vi "Tetra_PROD_Instruments.vi"(8 "error in":errorcluster) -> (1 "error out":errorcluster, 3 "This VI":refnum<vi>)   [LabVIEW 2018]
uses:
  <vilib>/Utility/error.llb/DialogType.ctl
  Initialize References/Sequence Globals.vi
  <vilib>/Utility/file.llb/Read Delimited Spreadsheet (string).vi
  Initialize References/Station References Global.vi
  Tetra_Globals.vi
  Instruments/Keysight N9010A/Agilent MXA Series/Agilent MXA Series.lvlib
  Instruments/Agilent N5232A PNA-L/Labview Driver/Keysight PNA Series/Keysight PNA Series.lvlib
panel:
  out "SN_LIST":string[][](array[string])
  out "selected comport":string
  out "USB toSER Present?":bool=TRUE
  out "find list":string[](array[string])
  in  "InitInterface(t)":bool=TRUE
  in  "InitGPIB(t)":bool=TRUE
  out "Test Station Information":string[](array[string])=["", "#INST: PS1#Address TCPIP0::169.254.70.130::inst0::INSTR#Manufacturer Agilent Technologies#Model N6700B#SN MY53000495#Ver D.02.01\n", "#INST: EXA#Address TCPIP0::169.254.70.120::inst0::INSTR#Manufacturer Keysight Technologies#Model N9010B#SN MY57470396#Ver A.27.05\n", "#INST: SigGen1#Address TCPIP0::169.254.70.100::inst0::INSTR#Manufacturer Agilent Technologies#Model N5173B#SN  MY53270534#Ver  B.01.95\n", "#INST: PNA#Address TCPIP0::169.254.70.180::inst0::INSTR#Manufacturer Agilent Technologies#Model N5232A#SN US52120122#Ver A.10.65.16\n", "#INST: RFSwitch#Address GPIB0::29::INSTR#Manufacturer AGILENT TECHNOLOGIES#Model 11713B#SN  MY52110609#Ver  A.01.08\n", "#INST: Gantry#Address COM5#Manufacturer Zaber#Model X-MCC4 (rev 1)#SN 81246#Ver (FW) 7.21 (DR) 1.5"]
  out "SigGen1Present?":bool=TRUE
  out "UseSigGen1(t)":bool=TRUE
  out "UsePS1(t)":bool=TRUE
  out "Use RFSwitch(t)":bool=TRUE
  out "Use SpecAn(t)":bool=TRUE
  out "Use PNA(t)":bool=TRUE
  out "Use Gantry(t)":bool=TRUE
  out "Use Oven(t)":bool
  out "Gantry Present?":bool=TRUE
  out "Array":errorcluster[](array[cluster])=[{"status"=FALSE, "code"=0, "source"=""}, {"status"=FALSE, "code"=0, "source"=""}, {"status"=FALSE, "code"=0, "source"=""}, {"status"=FALSE, "code"=0, "source"=""}, {"status"=FALSE, "code"=0, "source"=""}, {"status"=FALSE, "code"=0, "source"=""}, {"status"=FALSE, "code"=1073481728, "source"="Zaber A Series.lvlib:Error Query.vi<ERR>\nInstrument 01 0 reports 1 warnings:  NC\r\n\r\n For warning explanations visit http://www.zaber.com/wiki/Manuals/ASCII_Protocol_Manual#Warning_Flags. \n\n\n<b>Complete call chain:</b>\r\n     Zaber A Series.lvlib:Error Query.vi\r\n     Zaber A Series.lvlib:Send Command.vi\r\n     Gantry_Read-Write.vi\r\n     Discover Gantry.vi\r\n     Tetra_PROD_Instruments.vi"}]
  in  "y":bool
  out "Instrument File":path=path "C:/RageATE/Automated Tests/Tetra WAM/PRODUCTION/Test Benches/Common/WAM_PROD_TEST_Instruments.csv"
  out "Use":bool[](array[boolean])=[FALSE, TRUE, TRUE, TRUE, TRUE, TRUE, TRUE]
  out "path":string="C:\\RageATE\\Automated Tests\\Tetra WAM\\PRODUCTION\\Test Benches\\Common\\WAM_PROD_TEST_Instruments.csv"
  out "RF Switch Present?":bool=TRUE
  out "Spectrum Analyzer Present?":bool=TRUE
  out "PNA Present?":bool=TRUE
  out "concatenated string":string="#Not Used\r#INST: PS1#Address TCPIP0::169.254.70.130::inst0::INSTR#Manufacturer Agilent Technologies#Model N6700B#SN MY53000495#Ver D.02.01#Present!!\r#INST: EXA#Address TCPIP0::169.254.70.120::inst0::INSTR#Manufacturer Keysight Technologies#Model N9010B#SN MY57470396#Ver A.27.05#Present!!\r#INST: SigGen1#Address TCPIP0::169.254.70.100::inst0::INSTR#Manufacturer Agilent Technologies#Model N5173B#SN  MY53270534#Ver  B.01.95#Present!!\r#INST: PNA#Address TCPIP0::169.254.70.180::inst0::INSTR#Manufacturer Agilent Technologies#Model N5232A#SN US52120122#Ver A.10.65.16#Present!!\r#INST: RFSwitch#Address GPIB0::29::INSTR#Manufacturer AGILENT TECHNOLOGIES#Model 11713B#SN  MY52110609#Ver  A.01.08#Present!!\r#INST: Gantry#Address COM5#Manufacturer Zaber#Model X-MCC4 (rev 1)#SN 81246#Ver (FW) 7.21 (DR) 1.5#Present!!\r"
  out "Oven Present?":bool
  out "PS1 Present?":bool=TRUE
  # "Inst File selected"
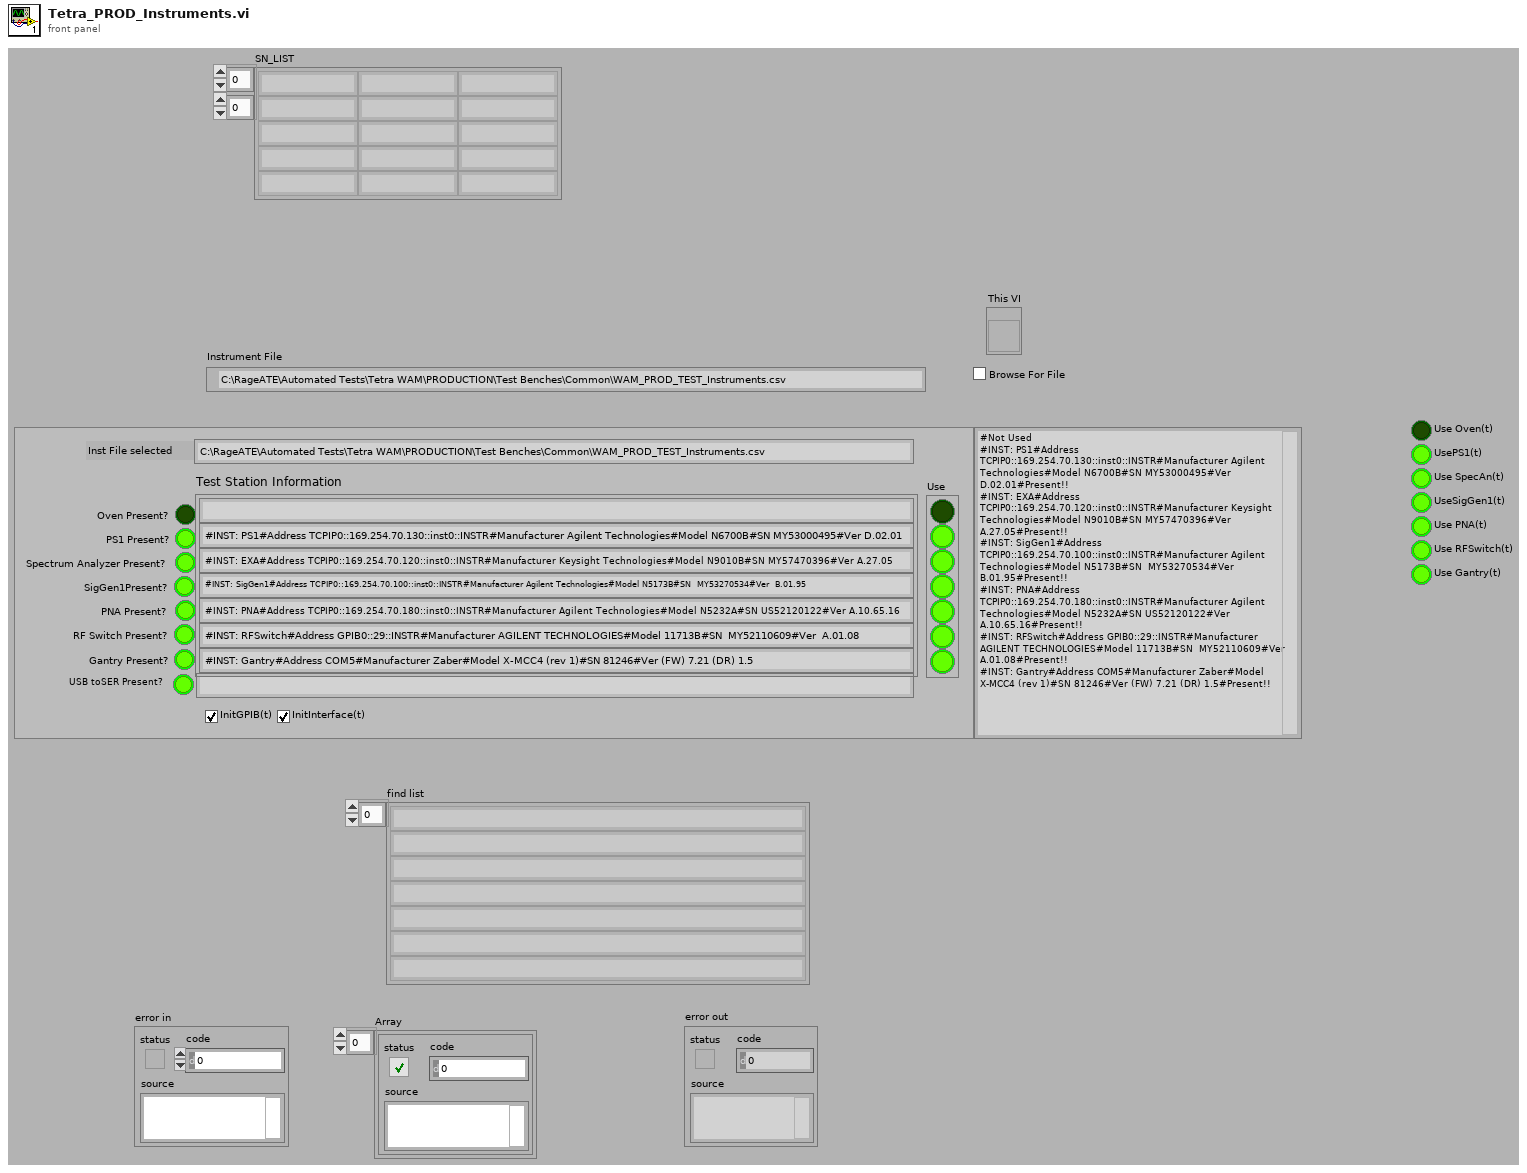
[diagram p1: front panel]
types:
  T1 = typedef "DialogType.ctl" = u16
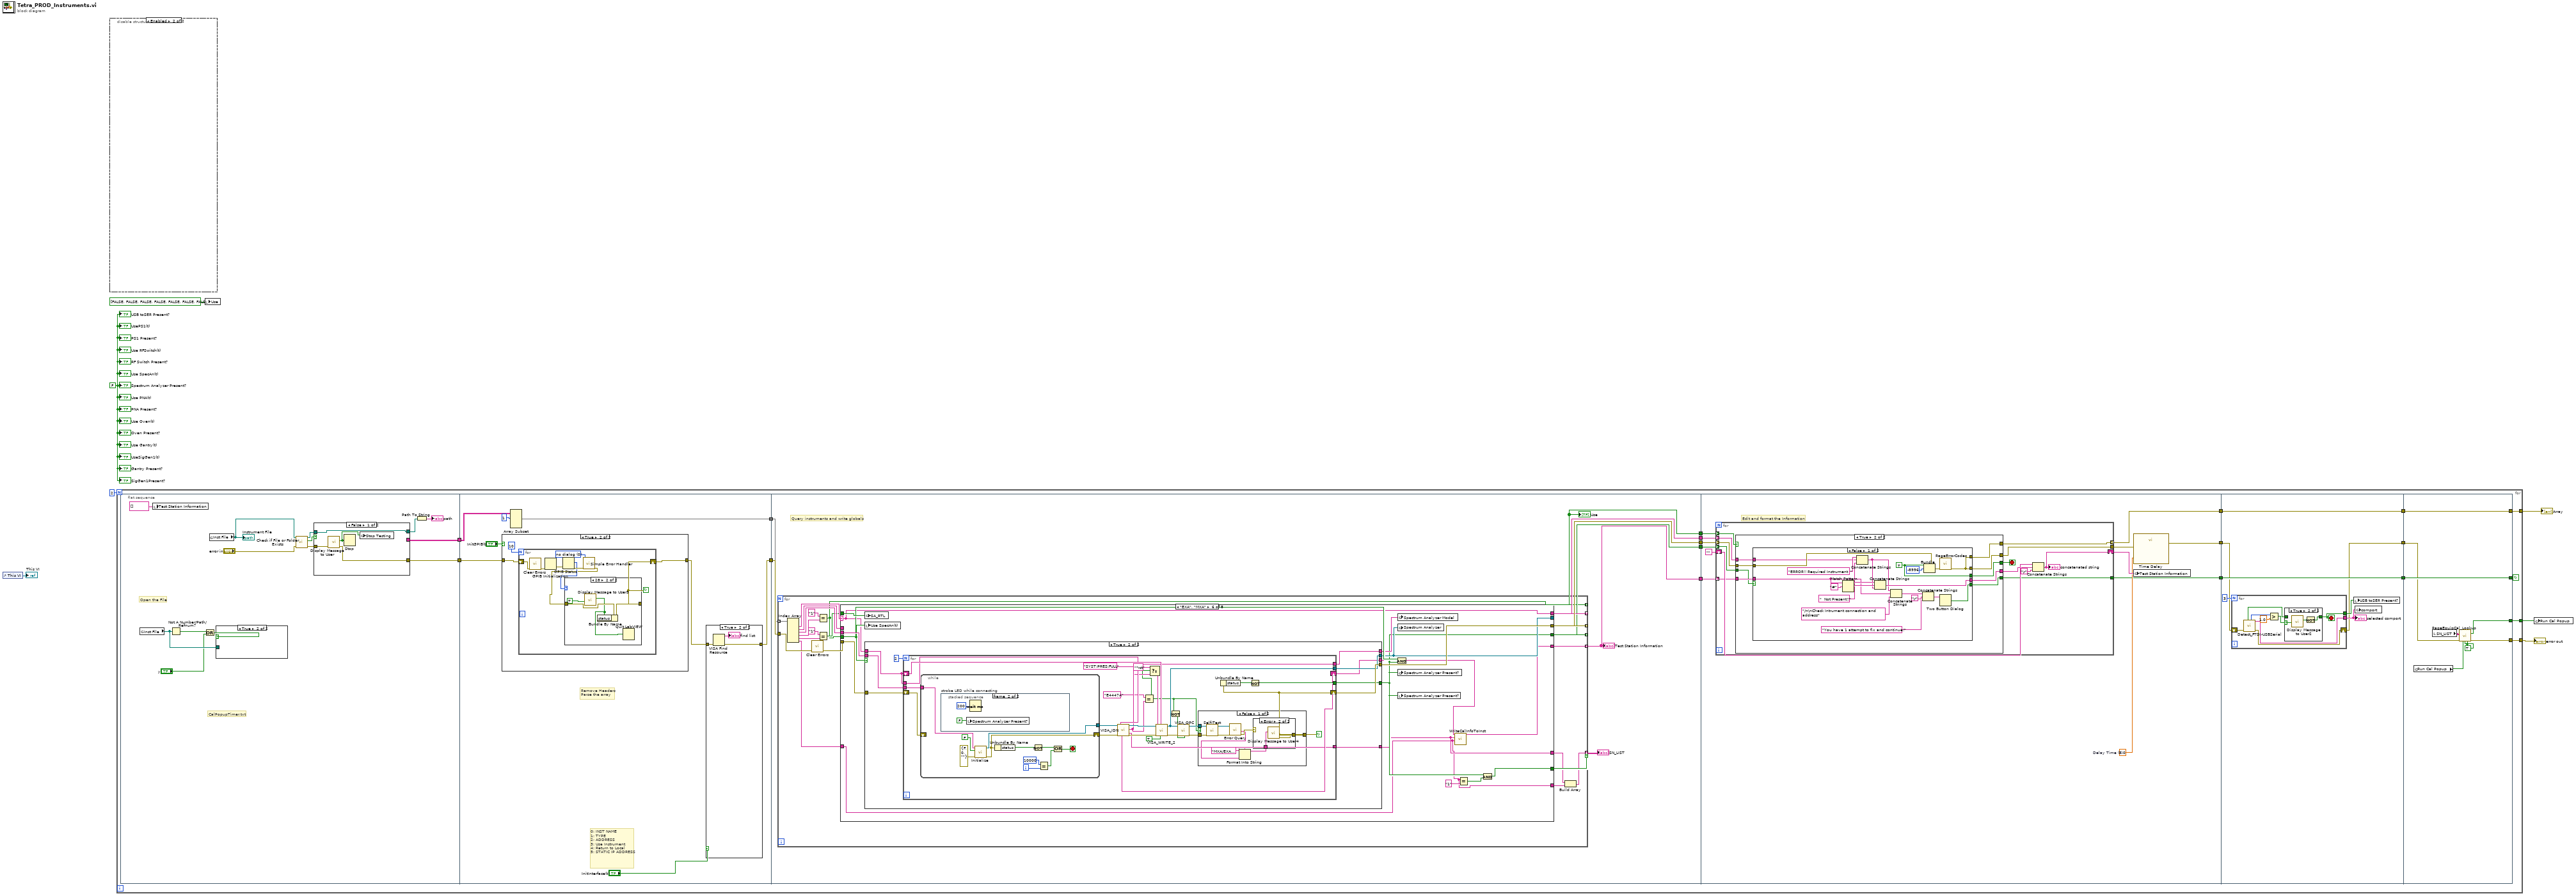
[diagram p0: block diagram]
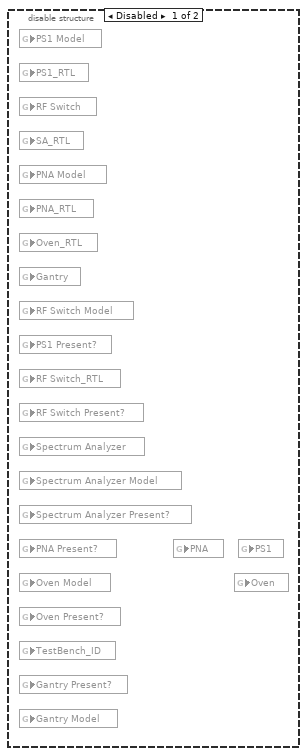
[diagram p2: hidden frame]
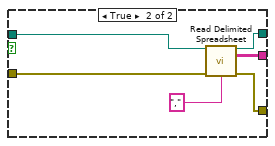
[diagram p4: hidden frame]
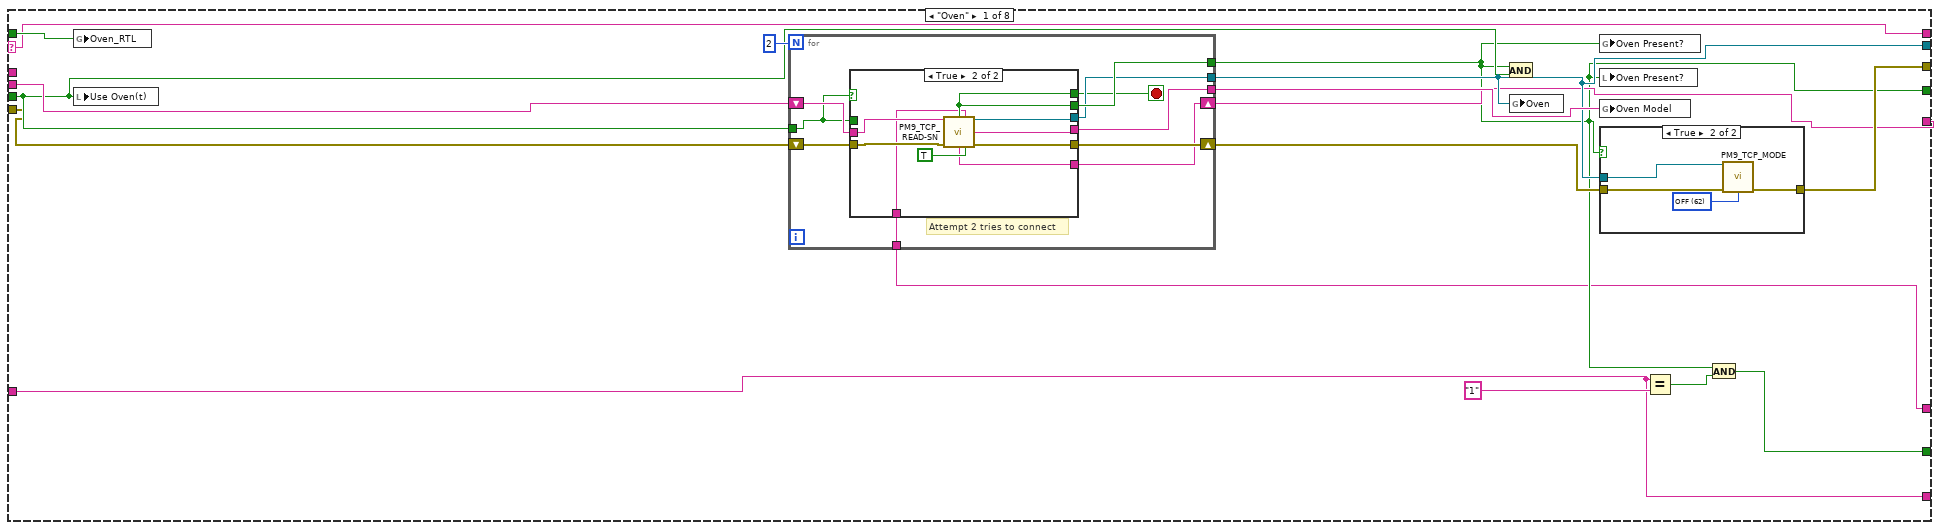
[diagram p8: hidden frame]
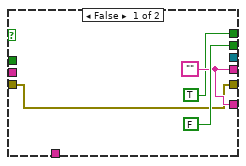
[diagram p10: hidden frame]
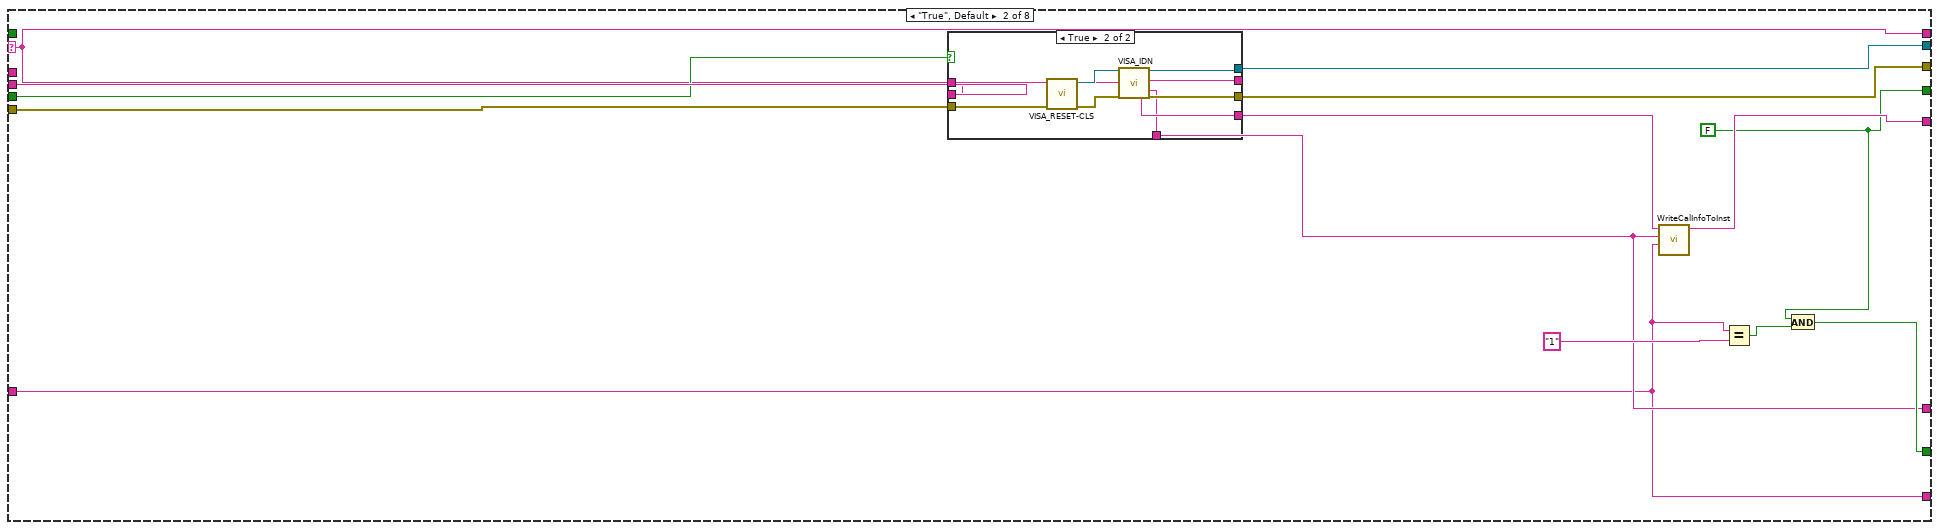
[diagram p11: hidden frame]
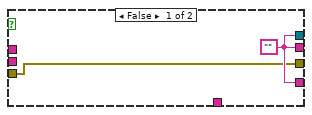
[diagram p12: hidden frame]
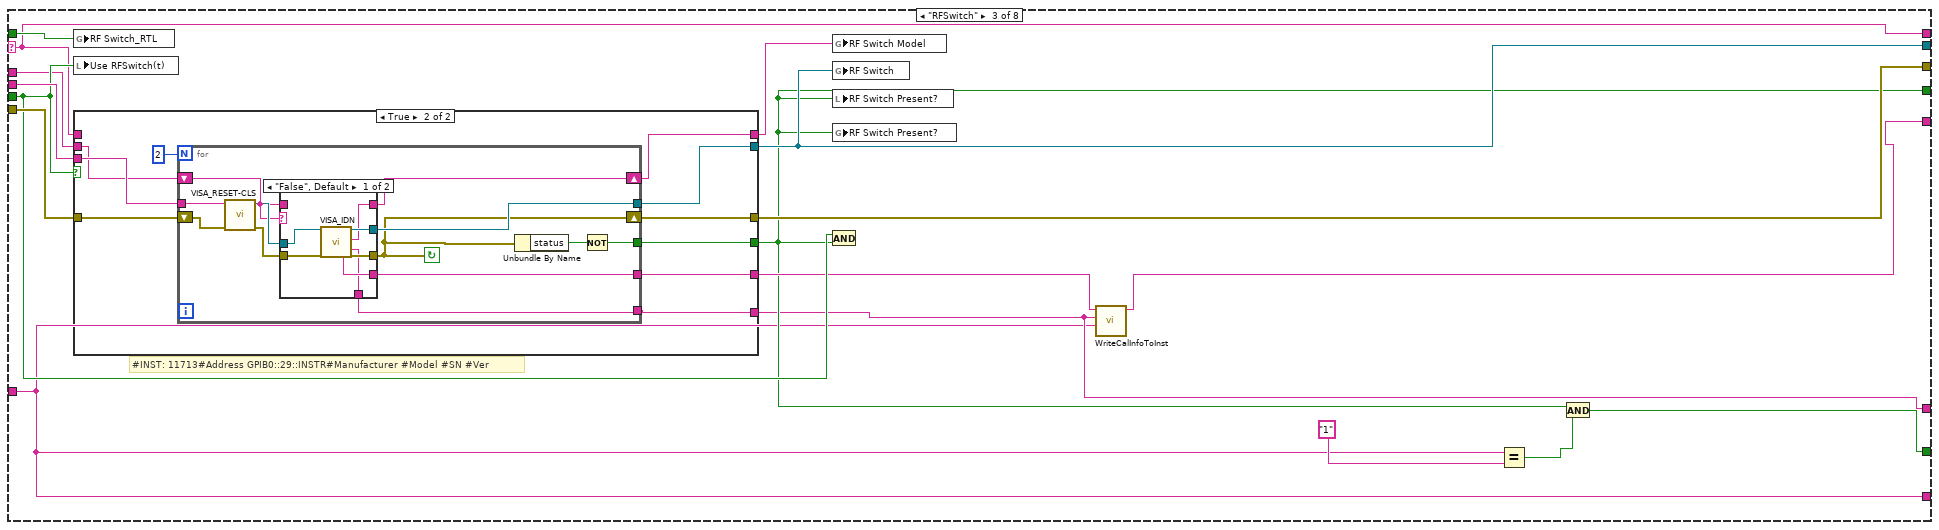
[diagram p13: hidden frame]
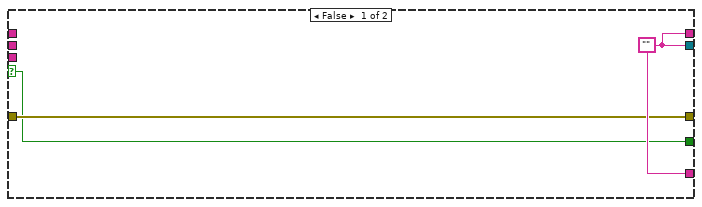
[diagram p14: hidden frame]
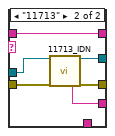
[diagram p15: hidden frame]
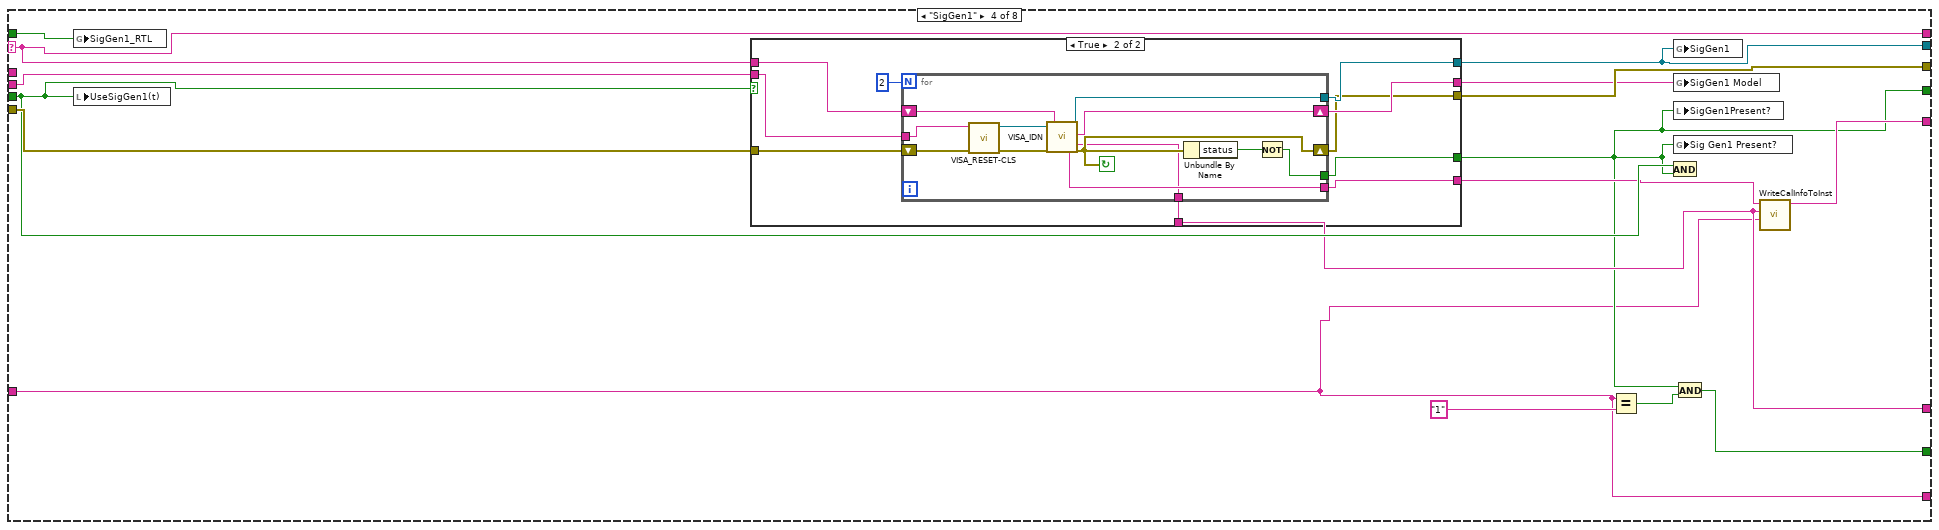
[diagram p16: hidden frame]
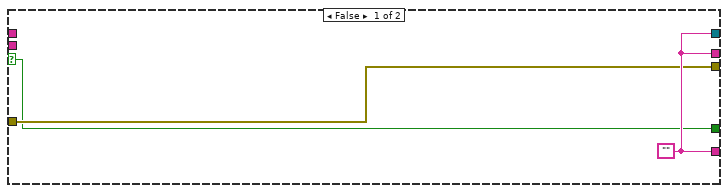
[diagram p17: hidden frame]
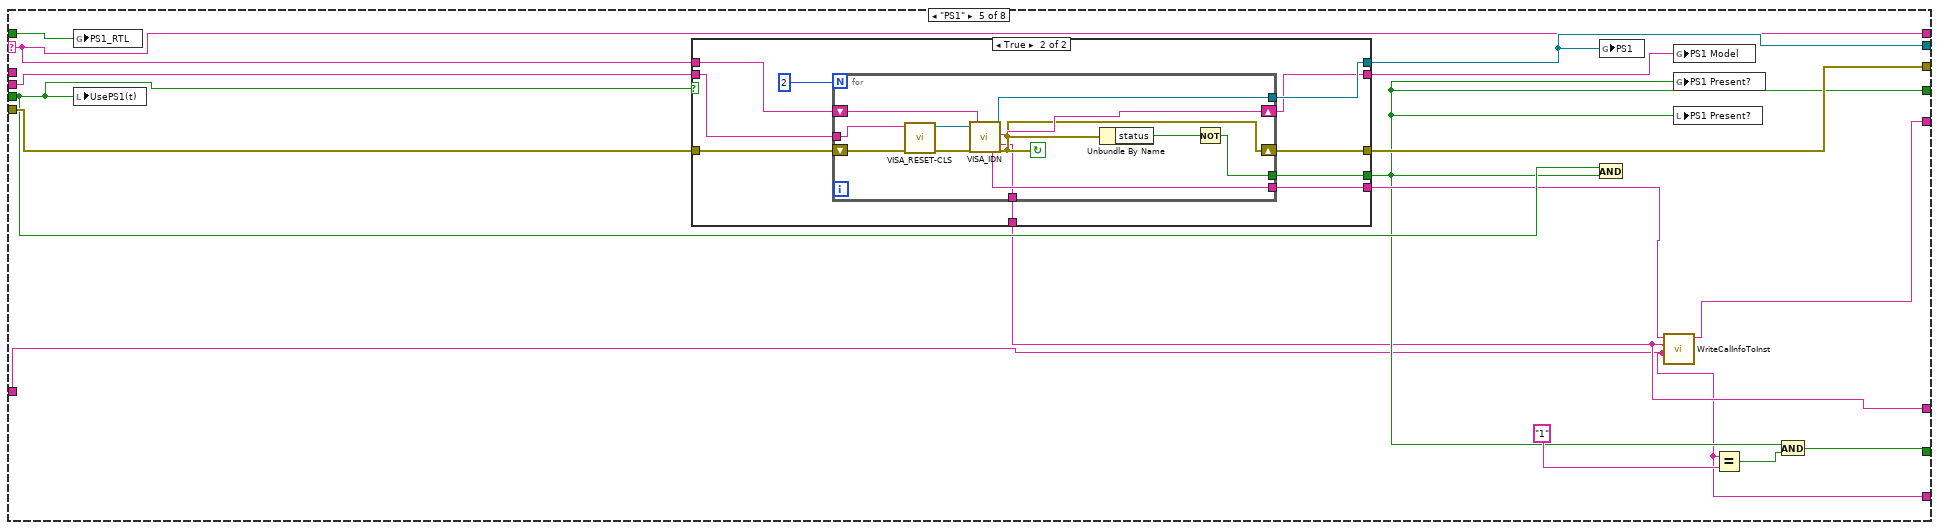
[diagram p18: hidden frame]
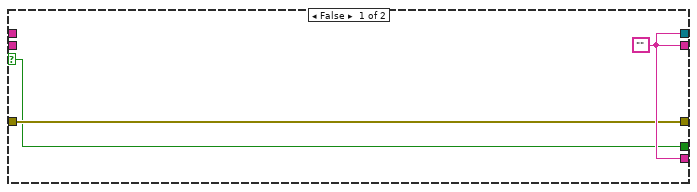
[diagram p19: hidden frame]
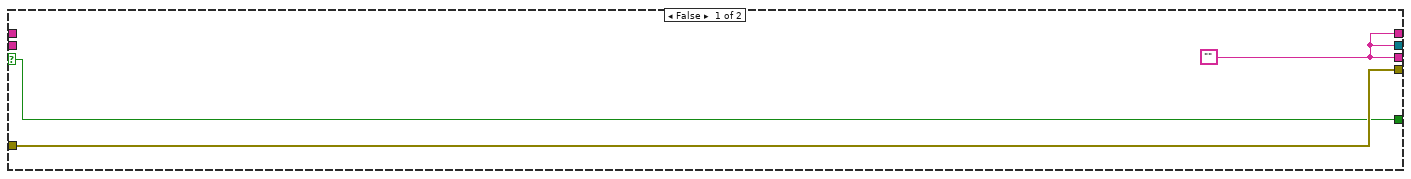
[diagram p20: hidden frame]
diagram:
  w4 = FALSE
  n1 = control-ref of="This VI"() -> (→"This VI":refnum<vi>)
  n2 = disable-structure shown="Enabled" {
    frame Disabled {
      n3 = global read "Station References Global.vi" "PS1 Model"() -> ()  [unwired: 1 in]
      n4 = global read "Station References Global.vi" "PS1_RTL"() -> ()  [unwired: 1 in]
      n5 = global read "Station References Global.vi" "RF Switch"() -> ()  [unwired: 1 in]
      n6 = global read "Station References Global.vi" "SA_RTL"() -> ()  [unwired: 1 in]
      n7 = global read "Station References Global.vi" "PNA Model"() -> ()  [unwired: 1 in]
      n8 = global read "Station References Global.vi" "PNA_RTL"() -> ()  [unwired: 1 in]
      n9 = global read "Station References Global.vi" "Oven_RTL"() -> ()  [unwired: 1 in]
      n10 = global read "Station References Global.vi" "Gantry"() -> ()  [unwired: 1 in]
      n11 = global read "Station References Global.vi" "RF Switch Model"() -> ()  [unwired: 1 in]
      n12 = global read "Station References Global.vi" "PS1 Present?"() -> ()  [unwired: 1 in]
      n13 = global read "Station References Global.vi" "RF Switch_RTL"() -> ()  [unwired: 1 in]
      n14 = global read "Station References Global.vi" "RF Switch Present?"() -> ()  [unwired: 1 in]
      n15 = global read "Station References Global.vi" "Spectrum Analyzer"() -> ()  [unwired: 1 in]
      n16 = global read "Station References Global.vi" "Spectrum Analyzer Model"() -> ()  [unwired: 1 in]
      n17 = global read "Station References Global.vi" "Spectrum Analyzer Present?"() -> ()  [unwired: 1 in]
      n18 = global read "Station References Global.vi" "PNA Present?"() -> ()  [unwired: 1 in]
      n19 = global read "Station References Global.vi" "Oven Model"() -> ()  [unwired: 1 in]
      n20 = global read "Station References Global.vi" "Oven Present?"() -> ()  [unwired: 1 in]
      n21 = global read "Tetra_Globals.vi" "TestBench_ID"() -> ()  [unwired: 1 in]
      n22 = global read "Station References Global.vi" "Gantry Present?"() -> ()  [unwired: 1 in]
      n23 = global read "Station References Global.vi" "Gantry Model"() -> ()  [unwired: 1 in]
      n24 = global read "Station References Global.vi" "PNA"() -> ()  [unwired: 1 in]
      n25 = global read "Station References Global.vi" "Oven"() -> ()  [unwired: 1 in]
      n26 = global read "Station References Global.vi" "PS1"() -> ()  [unwired: 1 in]
    }
    frame Enabled {
    }
  }
  n27 = for {
    N: 2 -> [_]
    tunnel: [w21] -> w7
    tunnel: [w9] -> w2
    tunnel: [w8] -> w1
    stop <- w20 continue-if-true
    n28 = flat-sequence {
      tunnel: [w38] -> w26
      tunnel: [w40] -> w25
      tunnel: [w51] -> w24
      tunnel: w26 -> [w55]
      tunnel: w25 -> [w57]
      tunnel: [w56] -> w19
      tunnel: w24 -> [w87]
      tunnel: [w86] -> w23
      tunnel: [w85] -> w22
      tunnel: w19 -> [w84]
      tunnel: [w83] -> w18
      tunnel: [w82] -> w17
      tunnel: [w81] -> w16
      tunnel: w23 -> [w495]
      tunnel: w22 -> [w497]
      tunnel: w18 -> [w490]
      tunnel: w17 -> [w488]
      tunnel: w16 -> [w489]
      tunnel: [w494] -> w15
      tunnel: [w492] -> w14
      tunnel: [w491] -> w13
      tunnel: w15 -> [w575]
      tunnel: w14 -> [w570]
      tunnel: w13 -> [w574]
      tunnel: [w575] -> w12
      tunnel: [w569] -> w11
      tunnel: [w574] -> w10
      tunnel: [w594] -> w20
      tunnel: [w595] -> w21
      tunnel: w12 -> [w595]
      tunnel: w11 -> [w591]
      tunnel: w10 -> [w594]
      tunnel: [w590] -> w9
      tunnel: [w588] -> w8
      frame #0 {
        # "Open the File"
        # "CalPopupTimer.txt"
        n29 = global read "Sequence Globals.vi" "Inst File"() -> (w30:path)
        n30 = local write "Test Station Information"(string[] [] ("Test Station Information")) -> ()
        n31 = Not A Number/Path/Refnum?(number/path/refnum=w30) -> (NaN/Path/Refnum?=w29:bool)
        n32 = Or(x=w29, y="y") -> (x .or. y?=w28:bool)
        n33 = global read "Sequence Globals.vi" "Inst File"() -> (w31:path)
        "Instrument File" <- w31
        n34 = case shown="True" w28 {
          tunnel: w30 -> [_ _]
          frame False {
          }
          frame True {
          }
        }
        n35 = call <vilib>:"Check if File or Folder Exists.vi"("error in (no error)"="error in", "path"=w31) -> ("error out"=w35:errorcluster, "file or folder exists?"=w33:bool, "dup path"=w34:path)  [unwired: 7 in]
        n36 = case shown="False" w33 {
          tunnel: [_ w49] -> w40
          tunnel: [w42 w48] -> w38
          tunnel: w35 -> [w43 w47]
          tunnel: [w44 w46] -> w37
          tunnel: w34 -> [w44 w45]
          frame False {
            n37 = call "Display Message to User"("error in (no error)"=w43) -> ("error out"=w42:errorcluster, "OK"=w41:bool)  [unwired: 9 in]
            n38 = Stop(stop? (T)=w41) -> ()
            n39 = global write "Sequence Globals.vi" "Stop Testing"(w41) -> ()
          }
          frame True {
            n40 = call-poly <vilib>:"Read Delimited Spreadsheet.vi"("file path (dialog if empty)"=w45, "error in (no error)"=w47, "delimiter (\\t)"="," ("delimiter (\\t)")) -> ("new file path (Not A Path if cancelled)"=w46:path, "all rows"=w49:string[][], "error out"=w48:errorcluster)  [unwired: 7 in, 3 out]
          }
        }
        n41 = Path To String(path=w37) -> (string=→"path":string)
      }
      frame #1 {
        # "0: INST NAME\n1: TYPE\n2: ADDRESS\n3: Use Instrument\n4: Return to Local\n5: STATIC IP ADDRESS"
        # "Remove Headers\nParse the array"
        n42 = case shown="True" "InitGPIB(t)" {
          tunnel: w55 -> [w63 w66]
          tunnel: [w63 w65] -> w52
          frame False {
          }
          frame True {
            n43 = for {
              N: 10 -> [_]
              shift-right: [w68] -> w65
              shift-left: w66 -> [w73]
              stop <- w68 continue-if-true
              w67 = T1 0 items=["no dialog", "OK message", "continue or stop message", "OK message + warnings", "continue/stop + warnings"] ("type of dialog (OK msg:1)")
              n44 = call <vilib>:"Clear Errors.vi"("error in (no error)"=w73) -> ("error out"=w74:errorcluster)  [unwired: 5 in, 1 out]
              n45 = GPIB Initialization(4:w74) -> (0:w72:errorcluster)  [unwired: 6 in]
              n46 = GPIB Status(1:w72) -> (3:w70:i16, 5:w71:errorcluster)  [unwired: 1 in, 2 out]
              n47 = call <vilib>:"Simple Error Handler.vi"("type of dialog (OK msg:1)"=w67, "error in (no error)"=w71) -> ("error out"=w69:errorcluster)  [unwired: 3 in, 4 out]
              n48 = case shown="28" w70 {
                tunnel: w69 -> [w75 w78]
                tunnel: [w75 w77] -> w68
                frame 0, Default {
                }
                frame 28 {
                  n49 = call "Display Message to User3"("Enable"=TRUE) -> ("OK (End)"=w76:bool)  [unwired: 9 in, 1 out]
                  n50 = Bundle By Name(cluster=w78, "status"=w76) -> (w77:errorcluster)
                  n51 = Quit LabVIEW(quit? (T)=w76) -> ()
                }
              }
            }
          }
        }
        n52 = Array Subset(array=w57, index (row)=1 ("index")) -> (w56:string[][])  [unwired: 3 in]
        n53 = case shown="True" "InitInterface(t)" {
          tunnel: w52 -> [w59 w61]
          tunnel: [w59 w62] -> w51
          frame False {
          }
          frame True {
            n54 = VISA Find Resource(8:w61) -> (0:w62:errorcluster, 3:→"find list":string[])  [unwired: 2 in, 1 out]
          }
        }
      }
      frame #2 {
        # "Query instruments and write globals"
        n55 = for {
          tunnel: w87 -> [w108]
          tunnel: [w96] -> w86 mode=indexing
          tunnel: [w95] -> w85 mode=indexing
          tunnel: w84 -> [w107] mode=indexing
          tunnel: [w98] -> w81 mode=indexing
          tunnel: [w97] -> w83 mode=indexing
          tunnel: [w94] -> w82 mode=indexing
          tunnel: [w89] -> w80 mode=indexing if=w91
          n56 = Index Array(array=w107) -> (element #1=w106:string, element #2=w104:string, element #3=w105:string, element #4=w102:string, element #5=w100:string, element #6=w92:string)  [unwired: 6 in]
          n57 = call <vilib>:"Clear Errors.vi"("error in (no error)"=w108) -> ("error out"=w93:errorcluster)  [unwired: 5 in, 1 out]
          n58 = Equal?(x="1", y=w102) -> (x = y?=w94:bool)
          n59 = Equal?(x="1", y=w100) -> (x = y?=w99:bool)
          n60 = case shown="\"EXA\", \"MXA\"" w106 {
            selector: w106 -> [w120 w162 w189 w243 w284 w325 w407 w445]
            tunnel: w93 -> [w116 w167 w196 w250 w291 w332 w414 w452]
            tunnel: [w119 w166 w193 w247 w288 w327 w409 w449] -> _
            tunnel: [w120 w162 w189 w243 w284 w325 w407 w445] -> w95
            tunnel: [w115 w160 w186 w242 w282 w323 w405 w443] -> w98
            tunnel: w105 -> [w125 w165 w195 w249 w290 w331 w412 w451]
            tunnel: w104 -> [_ _ w188 _ _ _ _ _]
            tunnel: w99 -> [w124 _ w192 w246 w287 w329 _ w447]
            tunnel: w94 -> [w122 w163 w190 w244 w285 w328 w411 w450]
            tunnel: [w111 w158 w183 w236 w278 w320 w400 w441] -> w97
            tunnel: [w117 w164 w194 w248 w289 w330 w410 w446] -> w96
            tunnel: w92 -> [w109 w154 w180 w235 w276 w317 w399 w437]
            tunnel: [w110 w155 w181 w238 w277 w318 w404 w442] -> w90
            tunnel: [w112 w156 w182 w237 w279 w319 w401 w439] -> w91
            tunnel: [w109 w154 w180 w235 w276 w317 w399 w437] -> w88
            frame "Oven" {
              n61 = global write "Station References Global.vi" "Oven_RTL"(w124) -> ()
              n62 = local write "Use Oven(t)"(w122) -> ()
              n63 = for {
                N: 2 -> [_]
                tunnel: w122 -> [w133]
                shift-right: [w139] -> w118
                shift-left: w116 -> [w140]
                shift-right: [w138] -> w115
                shift-left: w125 -> [w137]
                tunnel: [w136] -> w111
                tunnel: [w135] -> w121
                tunnel: [w134] -> w119
                tunnel: [w131] -> w110
                stop <- w132 stop-if-true
                # "Attempt 2 tries to connect"
                n64 = case shown="True" w133 {
                  tunnel: w140 -> [w142 w153]
                  tunnel: [w142 w151] -> w139
                  tunnel: [w143 w150] -> w138
                  tunnel: [_ w149] -> w134
                  tunnel: w137 -> [_ w148]
                  tunnel: [w143 w147] -> w135
                  tunnel: [FALSE ("selection") w146] -> w136
                  tunnel: w133 -> [_ _]
                  tunnel: [TRUE w146] -> w132
                  tunnel: [_ w145] -> w131
                  frame False {
                    w143 = ""
                  }
                  frame True {
                    n65 = call "PM9_TCP_READ-SN.vi"("VISA"=w148, "error in (no error)"=w153, "Close tcp(t)"=TRUE) -> ("Dev OK(t)"=w146:bool, "SN"=w145:string, "visa out"=w149:refnum<visa-resource-name>, "Model"=w147:string, "Device Info"=w150:string, "error out"=w151:errorcluster)  [unwired: 6 in, 1 out]
                  }
                }
              }
              n66 = And(x=w111, y=w122) -> ()  [unwired: 1 out]
              n67 = global write "Station References Global.vi" "Oven"(w119) -> ()
              n68 = global write "Station References Global.vi" "Oven Present?"(w111) -> ()
              n69 = local write "Oven Present?"(w111) -> ()
              n70 = global write "Station References Global.vi" "Oven Model"(w121) -> ()
              n71 = case shown="True" w111 {
                tunnel: w119 -> [_ w130]
                tunnel: w118 -> [w126 w129]
                tunnel: [w126 w128] -> w117
                frame False {
                }
                frame True {
                  w127 = u16 62 items=["READ ONLY"=0, "AUTO"=10, "OFF"=62, "MAN"=54] ("MODE")
                  n72 = call "PM9_TCP_MODE.vi"("VISA"=w130, "error in (no error)"=w129, "MODE"=w127) -> ("error out"=w128:errorcluster)  [unwired: 9 in, 3 out]
                }
              }
              n73 = Equal?(x=w109, y="1") -> (x = y?=w113:bool)
              n74 = And(x=w111, y=w113) -> (x .and. y?=w112:bool)
            }
            frame "True", Default {
              w158 = FALSE
              n75 = case shown="True" w163 {
                tunnel: w167 -> [w168 w179]
                tunnel: [w169 w177] -> w166
                tunnel: [w169 w176] -> _
                tunnel: [w169 w175] -> w161
                tunnel: w162 -> [_ w173]
                tunnel: w165 -> [_ w172]
                tunnel: [w168 w171] -> w164
                tunnel: [_ w170] -> w155
                frame False {
                  w169 = ""
                }
                frame True {
                  n76 = call "VISA_RESET-CLS.vi"("error in"=w179, "Session In"=w172) -> ("error out"=w178:errorcluster, "Session Out"=w174:refnum<visa-resource-name>)  [unwired: 8 in]
                  n77 = call "VISA_IDN.vi"("Session In"=w174, "error in"=w178, "INST(name)"=w173) -> ("concatenated string"=w175:string, "Session Out"=w177:refnum<visa-resource-name>, "Model"=w176:string, "SN"=w170:string, "error out"=w171:errorcluster)  [unwired: 10 in, 2 out]
                }
              }
              n78 = call "WriteCalInfoToInst.vi"("Enable"=w154, "SN"=w155, "TestInfo_In"=w161) -> ("TestInfo_Out"=w160:string)  [unwired: 8 in]
              n79 = Equal?(x=w154, y="1") -> (x = y?=w159:bool)
              n80 = And(x=w158, y=w159) -> (x .and. y?=w156:bool)
            }
            frame "RFSwitch" {
              # "#INST: 11713#Address GPIB0::29::INSTR#Manufacturer #Model #SN #Ver"
              n81 = global write "Station References Global.vi" "RF Switch_RTL"(w192) -> ()
              n82 = local write "Use RFSwitch(t)"(w190) -> ()
              n83 = case shown="True" w190 {
                selector: w190 -> [w197 _]
                tunnel: w196 -> [w198 w209]
                tunnel: [w199 w208] -> w193
                tunnel: [w199 w207] -> w191
                tunnel: [w199 w206] -> w187
                tunnel: [w198 w205] -> w194
                tunnel: w189 -> [_ _]
                tunnel: w195 -> [_ w204]
                tunnel: [w197 w202] -> w183
                tunnel: w188 -> [_ w201]
                tunnel: [_ w200] -> w181
                frame False {
                  w199 = ""
                }
                frame True {
                  n84 = for {
                    N: 2 -> [_]
                    tunnel: [w219] -> w208
                    tunnel: [w217] -> w206
                    tunnel: w204 -> [w215]
                    shift-right: [w214] -> w205
                    shift-left: w209 -> [w221]
                    shift-right: [w218] -> w207
                    shift-left: w201 -> [w211]
                    tunnel: [w212] -> w202
                    tunnel: [w210] -> w200
                    stop <- w214 continue-if-true
                    n85 = call "VISA_RESET-CLS.vi"("error in"=w221, "Session In"=w215) -> ("error out"=w220:errorcluster, "Session Out"=w216:refnum<visa-resource-name>)  [unwired: 8 in]
                    n86 = case shown="\"False\", Default" w211 {
                      tunnel: w220 -> [w228 w229]
                      tunnel: [w227 w232] -> w219
                      tunnel: [w223 w234] -> w218
                      tunnel: [w226 w231] -> w217
                      tunnel: w216 -> [w225 w233]
                      tunnel: w211 -> [_ w234]
                      tunnel: [w224 w230] -> w214
                      tunnel: [w222 _] -> w210
                      frame "False", Default {
                        n87 = call "VISA_IDN.vi"("Session In"=w225, "error in"=w228) -> ("concatenated string"=w226:string, "Session Out"=w227:refnum<visa-resource-name>, "Model"=w223:string, "SN"=w222:string, "error out"=w224:errorcluster)  [unwired: 11 in, 2 out]
                      }
                      frame "11713" {
                        n88 = call "11713_IDN.vi"("Session In"=w233, "error in"=w229) -> ("concatenated string"=w231:string, "Session Out"=w232:refnum<visa-resource-name>, "error out"=w230:errorcluster)  [unwired: 14 in, 1 out]
                      }
                    }
                    n89 = Unbundle By Name(w214) -> ("status"=w213:bool)
                    n90 = Not(x=w213) -> (.not. x?=w212:bool)
                  }
                }
              }
              n91 = And(x=w190, y=w183) -> ()  [unwired: 1 out]
              n92 = global write "Station References Global.vi" "RF Switch Model"(w191) -> ()
              n93 = global write "Station References Global.vi" "RF Switch"(w193) -> ()
              n94 = local write "RF Switch Present?"(w183) -> ()
              n95 = global write "Station References Global.vi" "RF Switch Present?"(w183) -> ()
              n96 = call "WriteCalInfoToInst.vi"("Enable"=w180, "SN"=w181, "TestInfo_In"=w187) -> ("TestInfo_Out"=w186:string)  [unwired: 8 in]
              n97 = Equal?(x=w180, y="1") -> (x = y?=w184:bool)
              n98 = And(x=w183, y=w184) -> (x .and. y?=w182:bool)
            }
            frame "SigGen1" {
              n99 = global write "Station References Global.vi" "SigGen1_RTL"(w246) -> ()
              n100 = local write "UseSigGen1(t)"(w244) -> ()
              n101 = case shown="True" w244 {
                selector: w244 -> [w251 _]
                tunnel: w250 -> [w252 w263]
                tunnel: [w253 w262] -> w247
                tunnel: [w253 w261] -> w245
                tunnel: [w253 w260] -> w241
                tunnel: [w252 w259] -> w248
                tunnel: w243 -> [_ w258]
                tunnel: w249 -> [_ w257]
                tunnel: [w251 w255] -> w236
                tunnel: [_ w254] -> w238
                frame False {
                  w253 = ""
                }
                frame True {
                  n102 = for {
                    N: 2 -> [_]
                    tunnel: [w273] -> w262
                    tunnel: [w271] -> w260
                    tunnel: w257 -> [w268]
                    shift-right: [w267] -> w259
                    shift-left: w263 -> [w275]
                    shift-right: [w272] -> w261
                    shift-left: w258 -> [w269]
                    tunnel: [w265] -> w255
                    tunnel: [w264] -> w254
                    stop <- w267 continue-if-true
                    n103 = call "VISA_RESET-CLS.vi"("error in"=w275, "Session In"=w268) -> ("error out"=w274:errorcluster, "Session Out"=w270:refnum<visa-resource-name>)  [unwired: 8 in]
                    n104 = call "VISA_IDN.vi"("Session In"=w270, "error in"=w274, "INST(name)"=w269) -> ("concatenated string"=w271:string, "Session Out"=w273:refnum<visa-resource-name>, "Model"=w272:string, "SN"=w264:string, "error out"=w267:errorcluster)  [unwired: 10 in, 2 out]
                    n105 = Unbundle By Name(w267) -> ("status"=w266:bool)
                    n106 = Not(x=w266) -> (.not. x?=w265:bool)
                  }
                }
              }
              n107 = Equal?(x=w235, y="1") -> (x = y?=w239:bool)
              n108 = And(x=w244, y=w236) -> ()  [unwired: 1 out]
              n109 = global write "Station References Global.vi" "SigGen1"(w247) -> ()
              n110 = global write "Station References Global.vi" "SigGen1 Model"(w245) -> ()
              n111 = local write "SigGen1Present?"(w236) -> ()
              n112 = global write "Station References Global.vi" "Sig Gen1 Present?"(w236) -> ()
              n113 = And(x=w236, y=w239) -> (x .and. y?=w237:bool)
              n114 = call "WriteCalInfoToInst.vi"("Enable"=w235, "SN"=w238, "TestInfo_In"=w241) -> ("TestInfo_Out"=w242:string)  [unwired: 8 in]
            }
            frame "PS1" {
              n115 = global write "Station References Global.vi" "PS1_RTL"(w287) -> ()
              n116 = local write "UsePS1(t)"(w285) -> ()
              n117 = case shown="True" w285 {
                selector: w285 -> [w292 _]
                tunnel: w291 -> [w293 w304]
                tunnel: [w294 w303] -> w288
                tunnel: [w294 w302] -> w286
                tunnel: [w294 w301] -> w283
                tunnel: [w293 w300] -> w289
                tunnel: w284 -> [_ w299]
                tunnel: w290 -> [_ w298]
                tunnel: [w292 w296] -> w278
                tunnel: [_ w295] -> w277
                frame False {
                  w294 = ""
                }
                frame True {
                  n118 = for {
                    N: 2 -> [_]
                    tunnel: [w314] -> w303
                    tunnel: [w312] -> w301
                    tunnel: w298 -> [w309]
                    shift-right: [w308] -> w300
                    shift-left: w304 -> [w316]
                    shift-right: [w313] -> w302
                    shift-left: w299 -> [w310]
                    tunnel: [w306] -> w296
                    tunnel: [w305] -> w295
                    stop <- w308 continue-if-true
                    n119 = call "VISA_RESET-CLS.vi"("error in"=w316, "Session In"=w309) -> ("error out"=w315:errorcluster, "Session Out"=w311:refnum<visa-resource-name>)  [unwired: 8 in]
                    n120 = call "VISA_IDN.vi"("Session In"=w311, "error in"=w315, "INST(name)"=w310) -> ("concatenated string"=w312:string, "Session Out"=w314:refnum<visa-resource-name>, "Model"=w313:string, "SN"=w305:string, "error out"=w308:errorcluster)  [unwired: 10 in, 2 out]
                    n121 = Unbundle By Name(w308) -> ("status"=w307:bool)
                    n122 = Not(x=w307) -> (.not. x?=w306:bool)
                  }
                }
              }
              n123 = And(x=w285, y=w278) -> ()  [unwired: 1 out]
              n124 = global write "Station References Global.vi" "PS1"(w288) -> ()
              n125 = call "WriteCalInfoToInst.vi"("Enable"=w276, "SN"=w277, "TestInfo_In"=w283) -> ("TestInfo_Out"=w282:string)  [unwired: 8 in]
              n126 = global write "Station References Global.vi" "PS1 Model"(w286) -> ()
              n127 = global write "Station References Global.vi" "PS1 Present?"(w278) -> ()
              n128 = local write "PS1 Present?"(w278) -> ()
              n129 = Equal?(x=w276, y="1") -> (x = y?=w280:bool)
              n130 = And(x=w278, y=w280) -> (x .and. y?=w279:bool)
            }
            frame "EXA", "MXA" {
              n131 = global write "Station References Global.vi" "SA_RTL"(w329) -> ()
              n132 = local write "Use SpecAn(t)"(w328) -> ()
              n133 = case shown="True" w328 {
                selector: w328 -> [w333 _]
                tunnel: w332 -> [w335 w345]
                tunnel: w331 -> [_ w340]
                tunnel: [w334 w343] -> w327
                tunnel: [w335 w344] -> w330
                tunnel: w325 -> [_ w337]
                tunnel: [w334 w342] -> w324
                tunnel: [w334 w341] -> w326
                tunnel: [w333 w338] -> w320
                tunnel: [_ w336] -> w318
                frame False {
                  w334 = ""
                }
                frame True {
                  n134 = for {
                    N: 2 -> [_]
                    tunnel: [w356] -> w343
                    tunnel: [w353] -> w341
                    tunnel: w340 -> [w363]
                    shift-right: [w358] -> w344
                    shift-left: w345 -> [w370]
                    shift-right: [w360] -> w342
                    shift-left: w337 -> [w364]
                    tunnel: [w361] -> w338
                    tunnel: w337 -> [w359]
                    tunnel: [w346] -> w336
                    stop <- w358 continue-if-true
                    n135 = while {
                      tunnel: w363 -> [w394]
                      tunnel: [w393] -> w369
                      shift-right: [w388] -> w367
                      shift-left: w370 -> [_]
                      i -> [w390]
                      stop <- w384 stop-if-true
                      n136 = stacked-sequence "strobe LED while connecting" {
                        frame #0 {
                          n137 = local write "Spectrum Analyzer Present?"(TRUE ("Spectrum Analyzer Present?")) -> ()
                          n138 = Wait (ms)(milliseconds to wait=u32 200) -> ()  [unwired: 1 out]
                        }
                        frame #1 {
                          n139 = local write "Spectrum Analyzer Present?"(FALSE ("Spectrum Analyzer Present?")) -> ()
                          n140 = Wait (ms)(milliseconds to wait=u32 200) -> ()  [unwired: 1 out]
                        }
                      }
                      n141 = call "Initialize.vi"("error in (no error)"=errorcluster {"status"=FALSE, "code"=0, "source"=""} ("error out"), "ID Query (True)"=FALSE, "VISA resource name"=w394) -> ("error out"=w388:errorcluster, "VISA resource name out"=w393:refnum<visa-resource-name>)  [unwired: 7 in]
                      n142 = Unbundle By Name(w388) -> ("status"=w386:bool)
                      n143 = Not(x=w386) -> (.not. x?=w385:bool)
                      n144 = Equal?(x=10000, y=w390) -> (x = y?=w387:bool)
                      n145 = Or(x=w385, y=w387) -> (x .or. y?=w384:bool)
                    }
                    n146 = call "VISA_IDN.vi"("Session In"=w369, "error in"=w367, "INST(name)"=w359) -> ("concatenated string"=w360:string, "Session Out"=w365:refnum<visa-resource-name>, "Model"=w353:string, "SN"=w346:string, "error out"=w366:errorcluster)  [unwired: 10 in, 2 out]
                    n147 = Equal?(x="E4447A", y=w353) -> (x = y?=w348:bool)
                    n148 = Select(t="*rst", s=w348, f="SYST:PRES:FULL" ("cmd")) -> (s? t:f=w351:string)
                    n149 = call "VISA_WRITE_2.vi"("No Value (T)"=TRUE, "Value (str)"=w364, "error in"=w366, "cmd"=w351, "Session In"=w365) -> ("error out"=w355:errorcluster, "Session Out"=w356:refnum<visa-resource-name>)  [unwired: 4 in, 1 out]
                    n150 = Not(x=w348) -> (.not. x?=w347:bool)
                    n151 = call "VISA_OPC.vi"("OPC(T)"=w347, "error in"=w355, "Session In"=w356) -> ("error out"=w354:errorcluster, "Session Out"=w357:refnum<visa-resource-name>)  [unwired: 6 in, 1 out]
                    n152 = case shown="False" w348 {
                      tunnel: [w374 w383] -> w358
                      tunnel: w357 -> [w379 _]
                      tunnel: w354 -> [w378 w383]
                      frame False {
                        n153 = call "Self-Test.vi"("error in (no error)"=w378, "VISA resource name"=w379) -> ("error out"=w376:errorcluster, "VISA resource name out"=w377:refnum<visa-resource-name>)  [unwired: 6 in, 2 out]
                        n154 = call "Error Query.vi"("error in (no error)"=w376, "VISA resource name"=w377) -> ("error out"=w375:errorcluster, "Error Message"=w371:string)  [unwired: 6 in, 2 out]
                        n155 = Format Into String(format string="MXA/EXA Reporting Errors :\n%s", w371) -> (resulting string=w372:string)  [unwired: 2 in, 1 out]
                        n156 = case shown="Error" w375 {
                          selector: w375 -> [w380 _]
                          tunnel: [w380 w382] -> w374
                          tunnel: w372 -> [_ w381]
                          frame No Error {
                          }
                          frame Error {
                            n157 = call "Display Message to User4"("Message"=w381) -> ("error out"=w382:errorcluster)  [unwired: 9 in, 1 out]
                          }
                        }
                      }
                      frame True {
                      }
                    }
                    n158 = Unbundle By Name(w358) -> ("status"=w362:bool)
                    n159 = Not(x=w362) -> (.not. x?=w361:bool)
                  }
                }
              }
              n160 = And(x=w328, y=w320) -> ()  [unwired: 1 out]
              n161 = global write "Station References Global.vi" "Spectrum Analyzer Model"(w326) -> ()
              n162 = global write "Station References Global.vi" "Spectrum Analyzer"(w327) -> ()
              n163 = global write "Station References Global.vi" "Spectrum Analyzer Present?"(w320) -> ()
              n164 = local write "Spectrum Analyzer Present?"(w320) -> ()
              n165 = call "WriteCalInfoToInst.vi"("Enable"=w317, "SN"=w318, "TestInfo_In"=w324) -> ("TestInfo_Out"=w323:string)  [unwired: 8 in]
              n166 = Equal?(x=w317, y="1") -> (x = y?=w321:bool)
              n167 = And(x=w320, y=w321) -> (x .and. y?=w319:bool)
            }
            frame "Gantry" {
              n168 = local write "Use Gantry(t)"(w411) -> ()
              n169 = case shown="True" w411 {
                tunnel: [w415 w427] -> w410
                tunnel: w414 -> [w415 w426]
                tunnel: [FALSE ("Gantry Present(t)") w425] -> w400
                tunnel: [w416 w424] -> w409
                tunnel: [w416 w423] -> w413
                tunnel: [w416 w422] -> w408
                tunnel: w411 -> [_ _]
                tunnel: w412 -> [_ w420]
                tunnel: [w416 w419] -> w406
                tunnel: [_ w418] -> w404
                frame False {
                  w416 = ""
                }
                frame True {
                  n170 = for {
                    N: 2 -> [_]
                    shift-right: [w436] -> w427
                    shift-left: w426 -> [w435]
                    tunnel: [w429] -> w425
                    tunnel: [w434] -> w424
                    tunnel: [w433] -> w423
                    tunnel: [w432] -> w422
                    tunnel: w420 -> [w431]
                    tunnel: [w430] -> w419
                    tunnel: [w428] -> w418
                    stop <- w429 stop-if-true
                    n171 = call "Discover Gantry.vi"("Session In"=w431, "error in"=w435) -> ("Gantry Present(t)"=w429:bool, "TestBench_ID"=w433:string, "concatenated string"=w430:string, "Session Out"=w434:refnum<visa-resource-name>, "Model"=w432:string, "SN"=w428:string, "error out"=w436:errorcluster)  [unwired: 9 in, 2 out]
                  }
                }
              }
              n172 = Equal?(x=w399, y="1") -> (x = y?=w402:bool)
              n173 = And(x=w400, y=w402) -> (x .and. y?=w401:bool)
              n174 = And(x=w400, y=w411) -> ()  [unwired: 1 out]
              n175 = local write "Gantry Present?"(w400) -> ()
              n176 = global write "Station References Global.vi" "Gantry Present?"(w400) -> ()
              n177 = global write "Tetra_Globals.vi" "TestBench_ID"(w413) -> ()
              n178 = global write "Station References Global.vi" "Gantry"(w409) -> ()
              n179 = global write "Station References Global.vi" "Gantry Model"(w408) -> ()
              n180 = call "WriteCalInfoToInst.vi"("Enable"=w399, "SN"=w404, "TestInfo_In"=w406) -> ("TestInfo_Out"=w405:string)  [unwired: 8 in]
            }
            frame "PNA" {
              n181 = global write "Station References Global.vi" "PNA_RTL"(w447) -> ()
              n182 = local write "Use PNA(t)"(w450) -> ()
              n183 = case shown="True" w450 {
                tunnel: [w454 w465] -> w449
                tunnel: [w454 w464] -> w448
                tunnel: [w455 w463] -> w446
                tunnel: [w454 w462] -> w444
                tunnel: w452 -> [w455 w461]
                tunnel: w451 -> [_ w460]
                tunnel: [FALSE w458] -> w441
                tunnel: w445 -> [_ w457]
                tunnel: [_ w456] -> w442
                frame False {
                  w454 = ""
                }
                frame True {
                  n184 = stacked-sequence "strobe LED while connecting" {
                    frame #0 {
                      n185 = local write "PNA Present?"(TRUE ("Spectrum Analyzer Present?")) -> ()
                      n186 = Wait (ms)(milliseconds to wait=u32 200) -> ()  [unwired: 1 out]
                    }
                    frame #1 {
                      n187 = local write "PNA Present?"(FALSE ("Spectrum Analyzer Present?")) -> ()
                      n188 = Wait (ms)(milliseconds to wait=u32 200) -> ()  [unwired: 1 out]
                    }
                  }
                  n189 = for {
                    N: 2 -> [_]
                    tunnel: [w487] -> w465
                    tunnel: [w486] -> w464
                    tunnel: [w485] -> w462
                    tunnel: w460 -> [w480]
                    shift-right: [w484] -> w463
                    shift-left: w461 -> [w479]
                    tunnel: [w482] -> w458
                    tunnel: w457 -> [w481]
                    tunnel: [w470] -> w456
                    stop <- w483 continue-if-true
                    w471 = 2 items=["Save", "Load", "Perform"] ("Action (0: Save)")
                    n190 = call "Initialize.vi"("error in (no error)"=w479, "Reset (True)"=FALSE, "VISA resource name"=w480) -> ("error out"=w474:errorcluster, "VISA resource name out"=w473:refnum<visa-resource-name>)  [unwired: 7 in]
                    n191 = call "Manage User Presets.vi"("error in (no error)"=w474, "Action (0: Save)"=w471, "VISA resource name"=w473) -> ("error out"=w475:errorcluster, "VISA resource name out"=w472:refnum<visa-resource-name>)  [unwired: 7 in]
                    n192 = call "Self-Test.vi"("error in (no error)"=w475, "VISA resource name"=w472) -> ("error out"=w478:errorcluster, "VISA resource name out"=w477:refnum<visa-resource-name>)  [unwired: 6 in, 2 out]
                    n193 = call "VISA_IDN.vi"("Session In"=w477, "error in"=w478, "INST(name)"=w481) -> ("concatenated string"=w485:string, "Session Out"=w487:refnum<visa-resource-name>, "Model"=w486:string, "SN"=w470:string, "error out"=w484:errorcluster)  [unwired: 10 in, 2 out]
                    n194 = Unbundle By Name(w484) -> ("status"=w483:bool)
                    n195 = Not(x=w483) -> (.not. x?=w482:bool)
                  }
                }
              }
              n196 = And(x=w450, y=w441) -> ()  [unwired: 1 out]
              n197 = global write "Station References Global.vi" "PNA"(w449) -> ()
              n198 = call "WriteCalInfoToInst.vi"("Enable"=w437, "SN"=w442, "TestInfo_In"=w444) -> ("TestInfo_Out"=w443:string)  [unwired: 8 in]
              n199 = global write "Station References Global.vi" "PNA Model"(w448) -> ()
              n200 = global write "Station References Global.vi" "PNA Present?"(w441) -> ()
              n201 = local write "PNA Present?"(w441) -> ()
              n202 = Equal?(x=w437, y="1") -> (x = y?=w438:bool)
              n203 = And(x=w441, y=w438) -> (x .and. y?=w439:bool)
            }
          }
          n204 = Build Array(w90, w88) -> (w89:string[])
        }
        "Test Station Information" <- w81
        "Use" <- w82
        "SN_LIST" <- w80
      }
      frame #3 {
        w496 = 2.0  # Delay Time (s)
        # "Edit and format the Information"
        n205 = for {
          tunnel: w497 -> [w500] mode=indexing
          shift-right: [w512] -> w499
          shift-left: "" -> [w511]
          tunnel: w490 -> [w510] mode=indexing
          tunnel: w495 -> [w509] mode=indexing
          tunnel: [w508] -> w494 mode=indexing
          tunnel: [w507] -> w493
          tunnel: [w505] -> w491
          tunnel: w488 -> [w502] mode=indexing
          tunnel: w489 -> [w501] mode=indexing
          stop <- w506 stop-if-true
          n206 = case shown="True" w502 {
            tunnel: w501 -> [w520 w541]
            tunnel: [w513 w540] -> w504
            tunnel: w510 -> [w519 w539]
            tunnel: w509 -> [w518 w538]
            tunnel: [w517 w537] -> w508
            tunnel: [errorcluster {"status"=FALSE, "code"=0, "source"=""} ("error out") w536] -> w507
            tunnel: [w515 w535] -> w506
            tunnel: [w515 w534] -> w505
            tunnel: w500 -> [_ w533]
            frame False {
              w515 = FALSE ("status")
              n207 = case shown="True" w519 {
                tunnel: w520 -> [w523 w531]
                tunnel: [w526 w530] -> w514
                tunnel: w518 -> [w525 w532]
                tunnel: [w525 w532] -> w517
                frame False {
                  n208 = call <vilib>:"Trim Whitespace.vi"("string"=w523) -> ("trimmed string"=w522:string)  [unwired: 1 in]
                  n209 = Concatenate Strings("#" ("string"), w522, "Not Used" ("string")) -> (w526:string)
                }
                frame True {
                  n210 = call <vilib>:"Trim Whitespace.vi"("string"=w531) -> ("trimmed string"=w528:string)  [unwired: 1 in]
                  n211 = Concatenate Strings("#" ("string"), w528, " Present but Not Used! " ("string")) -> (w530:string)
                }
              }
              n212 = call <vilib>:"Trim Whitespace.vi"("string"=w514) -> ("trimmed string"=w513:string)  [unwired: 1 in]
            }
            frame True {
              n213 = case shown="False" w539 {
                tunnel: w541 -> [w553 w564]
                tunnel: [w558 w568] -> w540
                tunnel: w538 -> [w556 w567]
                tunnel: [w550 w567] -> w537
                tunnel: [w550 errorcluster {"status"=FALSE, "code"=0, "source"=""} ("error out")] -> w536
                tunnel: [w549 w565] -> w535
                tunnel: [w545 w565] -> w534
                tunnel: w533 -> [w542 _]
                frame False {
                  w549 = TRUE ("status")
                  n214 = Match Pattern(string=w553, regular expression="#") -> (before substring=w560:string, match substring=w559:string)  [unwired: 1 in, 2 out]
                  n215 = Concatenate Strings("ERROR!! Required Instrument  " ("string"), w542, "  Not Present!!" ("string")) -> (w544:string)
                  n216 = Concatenate Strings(w560, w559, w544) -> (w558:string)
                  n217 = Concatenate Strings(w544, w553, "/n\nCheck Intrument connection and address" ("string")) -> (w552:string)
                  n218 = Concatenate Strings(w552, "\r", "You have 1 attempt to fix and continue!" ("string")) -> (w548:string)
                  n219 = Bundle(cluster=w556, "status"=w549, "code"=-8996) -> (w555:errorcluster)  [unwired: 1 in]
                  n220 = call "RageErrorCodes.vi"("error in"=w555) -> ("error out"=w550:errorcluster)  [unwired: 8 in, 2 out]
                  n221 = Two Button Dialog(message=w548) -> (T button?=w545:bool)  [unwired: 2 in]
                }
                frame True {
                  w565 = FALSE ("status")
                  n222 = call <vilib>:"Trim Whitespace.vi"("string"=w564) -> ("trimmed string"=w563:string)  [unwired: 1 in]
                  n223 = Concatenate Strings(w563, "#Present!!" ("string")) -> (w568:string)
                }
              }
            }
          }
          n224 = Concatenate Strings(w511, w504, "\r") -> (w512:string)
          "concatenated string" <- w512
        }
        n225 = call "Time Delay"("error in (no error)"=w493, "Delay Time (s)"=w496) -> ("error out"=w492:errorcluster)  [unwired: 9 in]
        n226 = global write "Station References Global.vi" "Test Station Information"(w499) -> ()
      }
      frame #4 {
        n227 = for {
          N: 3 -> [_]
          tunnel: [w581] -> w572
          tunnel: [w576] -> w573
          shift-right: [w583] -> w569
          shift-left: w570 -> [w582]
          stop <- w576 stop-if-true
          n228 = call "Detect_FTDI-USBSerial.vi"("error in (no error)"=w582) -> ("error out"=w583:errorcluster, "selected comport"=w581:string, "# of FTDI Devices"=w578:i32, "Success(t)"=w577:bool)  [unwired: 7 in]
          n229 = Greater?(x=w578, y=1.0) -> (0:w580:bool)
          n230 = case shown="True" w580 {
            selector: w580 -> [_ w585]
            tunnel: w577 -> [w584 _]
            tunnel: [w584 w586] -> w576
            frame False {
            }
            frame True {
              n231 = call "Display Message to User2"("Enable"=w585) -> ("OK"=w587:bool)  [unwired: 9 in, 1 out]
              n232 = Not(x=w587) -> (.not. x?=w586:bool)
            }
          }
        }
        "selected comport" <- w572
        n233 = local write "USB toSER Present?"(w573) -> ()
        n234 = global write "Tetra_Globals.vi" "comport"(w572) -> ()
      }
      frame #5 {
        w592 = TRUE ("Use Popup Warning(T)")
        n235 = global read "Station References Global.vi" "Run Cal Popup"() -> (w589:bool)
        n236 = local read "SN_LIST"() -> (w593:string[][])
        n237 = call "RageEquipCal_Lookup.vi"("SN / Active(1=T)"=w593, "error in (no error)"=w591, 12:"Use Popup Warning(T)"=w589, "Run Vi (T)"=w592, 14:"Use Popup Warning(T)"=w592) -> ("OK"=w588:bool, "error out"=w590:errorcluster)  [unwired: 8 in, 1 out]
      }
    }
  }
  "Array" <- w7
  "error out" <- w2
  n238 = local write "Use"(bool[] [FALSE, FALSE, FALSE, FALSE, FALSE, FALSE, FALSE] ("Use")) -> ()
  n239 = global write "Station References Global.vi" "Run Cal Popup"(w1) -> ()
  "Oven Present?" <- w4
  "Use Oven(t)" <- w4
  "Gantry Present?" <- w4
  "Use Gantry(t)" <- w4
  "PNA Present?" <- w4
  "Use PNA(t)" <- w4
  "Spectrum Analyzer Present?" <- w4
  "Use SpecAn(t)" <- w4
  "RF Switch Present?" <- w4
  "PS1 Present?" <- w4
  "Use RFSwitch(t)" <- w4
  "UsePS1(t)" <- w4
  "UseSigGen1(t)" <- w4
  "SigGen1Present?" <- w4
  "USB toSER Present?" <- w4
